vi "generate_frame.vi"(3 "error in (no error)":errorcluster, 4 "Frame number":i32, 5 "Frames":T1(array[cluster])) -> (0 "error out":errorcluster, 1 "Done":bool, 2 "Frame":string)   [LabVIEW 2019, in "Lib_Simx.lvlib"]
doc: "Obtains a frame from the array of frames and generates the JSON text to send to the simulator."
uses:
  Lib_Simx.lvlib
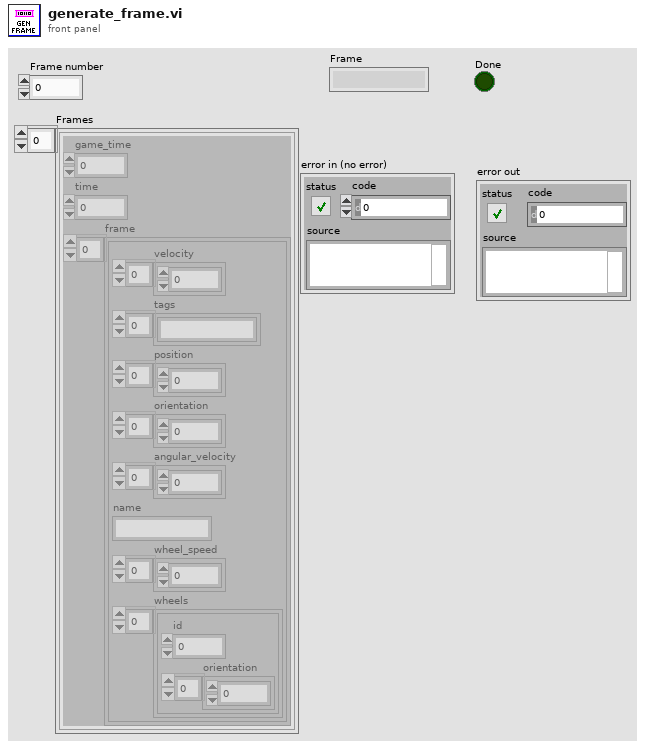
[diagram p1: front panel]
types:
  T1 = cluster{"game_time":dbl, "time":dbl, "frame":cluster{"velocity":dbl[], "tags":string[], "position":dbl[], "orientation":dbl[], "angular_velocity":dbl[], "name":string, "wheel_speed":dbl[], "wheels":cluster{"id":i32, "orientation":dbl[]}[]}[]}[]
  T2 = cluster{"game_time":dbl, "time":dbl, "frame":cluster{"velocity":dbl[], "tags":string[], "position":dbl[], "orientation":dbl[], "angular_velocity":dbl[], "name":string, "wheel_speed":dbl[], "wheels":cluster{"id":i32, "orientation":dbl[]}[]}[]}
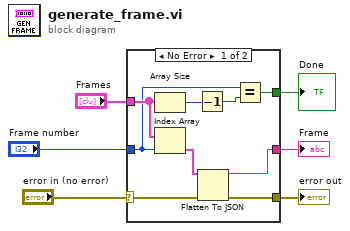
[diagram p0: block diagram]
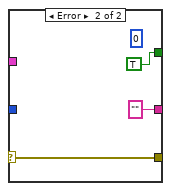
[diagram p2: hidden frame]
diagram:
  n1 = case shown="No Error" "error in (no error)" {
    selector: "error in (no error)" -> [w12 w18]
    tunnel: "Frames" -> [w15 _]
    tunnel: "Frame number" -> [w9 _]
    tunnel: [w13 "" ("JSON string")] -> w4
    tunnel: [w11 w18] -> w2
    tunnel: [w7 TRUE] -> w1
    frame No Error {
      n2 = Array Size(array=w15) -> (size(s)=w8:i32)
      n3 = Index Array(array=w15, index=w9) -> (element=w14:T2)
      n4 = Decrement(x=w8) -> (x-1=w10:i32)
      n5 = Flatten To JSON(anything=w14, error in (no error)=w12) -> (JSON string=w13:string, 11:w11:errorcluster)  [unwired: 1 in]
      n6 = Equal?(x=w9, y=w10) -> (x = y?=w7:bool)
    }
    frame Error {
      (unwired) 0
    }
  }
  "Frame" <- w4
  "error out" <- w2
  "Done" <- w1
